vi "AddIntake.vi"(10 "Intake out":bool, 11 "Refnum in":T1) -> (3 "Refnum out":T1)   [LabVIEW 2019]
uses:
  <vilib>/vision/Image Controls.llb/IMAQ Image.ctl
  <vilib>/vision/NI_Vision_Development_Module.lvlib
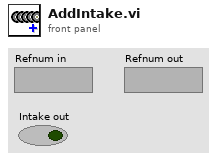
[diagram p1: front panel]
types:
  T1 = typedef "IMAQ Image.ctl" = refnum<image>
  T2 = typedef "Image Type" = u32
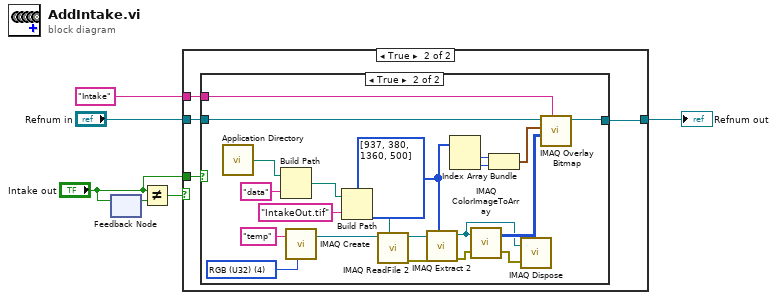
[diagram p0: block diagram]
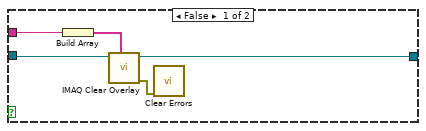
[diagram p3: hidden frame]
diagram:
  n1 = feedback-in #1("Intake out") -> ()
  n2 = feedback #1() -> (w5:bool)  [unwired: 1 in]
  n3 = Not Equal?(x="Intake out", y=w5) -> (x != y?=w6:bool)
  n4 = case shown="True" w6 {
    tunnel: [w7 w9] -> w4
    tunnel: "Refnum in" -> [w7 w10]
    tunnel: "Intake out" -> [_ w11]
    tunnel: "Intake" -> [_ w8]
    frame False {
    }
    frame True {
      n5 = case shown="True" w11 {
        tunnel: w10 -> [w16 w36]
        tunnel: [w15 w35] -> w9
        tunnel: w8 -> [w14 w37]
        frame False {
          n6 = Build Array(w14) -> (w13:string[])
          n7 = call "IMAQ Clear Overlay"("Groups"=w13, "Image"=w16) -> ("error out"=w12:errorcluster, "Image Out"=w15:T1)  [unwired: 8 in]
          n8 = call <vilib>:"Clear Errors.vi"("error in (no error)"=w12) -> ()  [unwired: 5 in, 2 out]
        }
        frame True {
          w22 = i32[] [937, 380, 1360, 500] ("Optional Rectangle")
          w28 = T2 4 items=["Grayscale (U8)", "Grayscale (I16)", "Grayscale (SGL)", "Complex (CSG)", "RGB (U32)", "HSL (U32)", "RGB (U64)", "Grayscale (U16)"] ("Image Type")
          n9 = call <vilib>:"Application Directory.vi"() -> ("Application Directory"=w33:path)
          n10 = Build Path(base path=w33, name or relative path="data") -> (appended path=w34:path)
          n11 = call "IMAQ Create"("Image Name"="temp", "Image Type"=w28) -> ("New Image"=w27:T1)  [unwired: 3 in, 1 out]
          n12 = Build Path(base path=w34, name or relative path="IntakeOut.tif") -> (appended path=w30:path)
          n13 = call "IMAQ ReadFile 2"("File Path"=w30, "Image"=w27) -> ("error out"=w26:errorcluster, "Image Out"=w25:T1)  [unwired: 5 in, 3 out]
          n14 = call "IMAQ Extract 2"("Optional Rectangle"=w22, "error in (no error)"=w26, "Image Src"=w25) -> ("error out"=w24:errorcluster, "Image Dst Out"=w17:T1)  [unwired: 7 in]
          n15 = Index Array(array=w22) -> (element #1=w20:i32, element #2=w21:i32)  [unwired: 2 in]
          n16 = call "IMAQ ColorImageToArray"("Image"=w17, "error in (no error)"=w24) -> ("Image Pixels (U32)"=w23:u32[][], "error out"=w18:errorcluster)  [unwired: 2 in, 1 out]
          n17 = Bundle(w20, w21) -> (w19:cluster{i32, i32})  [unwired: 1 in]
          n18 = call "IMAQ Dispose"("Image"=w17, "error in (no error)"=w18) -> ()  [unwired: 4 in, 1 out]
          n19 = call "IMAQ Overlay Bitmap"("Group"=w37, "Bitmap"=w23, "Top Left Point"=w19, "Image"=w36) -> ("Image Out"=w35:T1)  [unwired: 6 in, 1 out]
        }
      }
    }
  }
  "Refnum out" <- w4
